vi "Calculate Points of Line without diagonal.vi"(8 "Yf":i32, 9 "Yi":i32, 10 "Xf":i32, 11 "Xi":i32) -> (2 "Y Points":i32[](array[numeric]), 3 "X Points":i32[](array[numeric]))   [LabVIEW 2019, in "Day 5.lvlib"]
uses:
  Day 5.lvlib
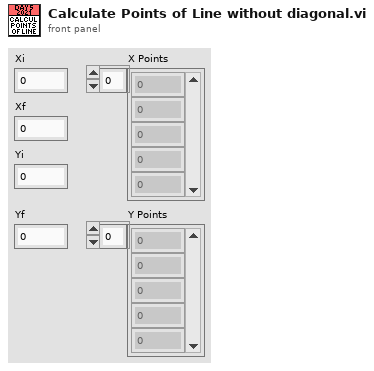
[diagram p1: front panel]
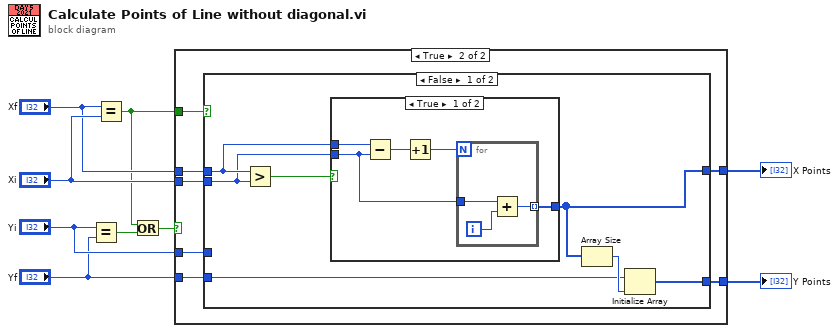
[diagram p0: block diagram]
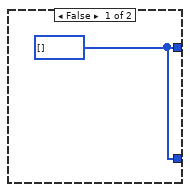
[diagram p2: hidden frame]
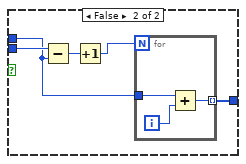
[diagram p3: hidden frame]
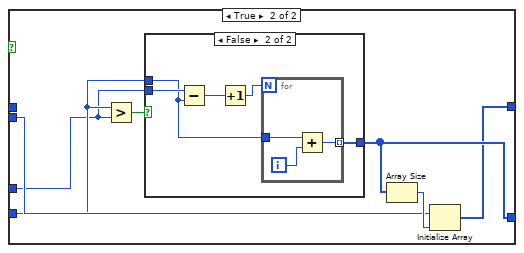
[diagram p4: hidden frame]
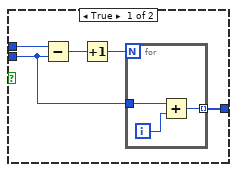
[diagram p5: hidden frame]
diagram:
  n1 = Equal?(x="Yi", y="Yf") -> (x = y?=w2:bool)
  n2 = Equal?(x="Xf", y="Xi") -> (x = y?=w3:bool)
  n3 = Or(x=w3, y=w2) -> (x .or. y?=w1:bool)
  n4 = case shown="True" w1 {
    tunnel: w3 -> [_ w17]
    tunnel: "Xi" -> [_ w16]
    tunnel: "Xf" -> [_ w15]
    tunnel: "Yi" -> [_ w14]
    tunnel: "Yf" -> [_ w13]
    tunnel: [w10 w12] -> w7
    tunnel: [w10 w11] -> w6
    frame False {
      w10 = i32[] []
    }
    frame True {
      n5 = case shown="False" w17 {
        tunnel: w16 -> [w22 w43]
        tunnel: w15 -> [w23 _]
        tunnel: w14 -> [_ w41]
        tunnel: w13 -> [w20 w42]
        tunnel: [w18 w46] -> w12
        tunnel: [w19 w44] -> w11
        frame False {
          n6 = Greater?(x=w23, y=w22) -> (0:w24:bool)
          n7 = case shown="True" w24 {
            tunnel: w23 -> [w29 w35]
            tunnel: w22 -> [w28 w36]
            tunnel: [w27 w37] -> w19
            frame True {
              n8 = Subtract(x=w29, y=w28) -> (x-y=w26:i32)
              n9 = Increment(x=w26) -> (x+1=w25:i32)
              n10 = for {
                N: w25 -> [_]
                tunnel: w28 -> [w32]
                tunnel: [w30] -> w27 mode=indexing
                i -> [w31]
                n11 = Add(x=w32, y=w31) -> (x+y=w30:i32)
              }
            }
            frame False {
              n12 = Subtract(x=w36, y=w35) -> (x-y=w34:i32)
              n13 = Increment(x=w34) -> (x+1=w33:i32)
              n14 = for {
                N: w33 -> [_]
                tunnel: w35 -> [w40]
                tunnel: [w38] -> w37 mode=indexing
                i -> [w39]
                n15 = Add(x=w40, y=w39) -> (x+y=w38:i32)
              }
            }
          }
          n16 = Array Size(array=w19) -> (size(s)=w21:i32)
          n17 = Initialize Array(w20, w21) -> (w18:i32[])
        }
        frame True {
          n18 = Greater?(x=w42, y=w41) -> (0:w47:bool)
          n19 = case shown="False" w47 {
            tunnel: w42 -> [w52 w58]
            tunnel: w41 -> [w51 w59]
            tunnel: [w50 w60] -> w46
            frame True {
              n20 = Subtract(x=w52, y=w51) -> (x-y=w49:i32)
              n21 = Increment(x=w49) -> (x+1=w48:i32)
              n22 = for {
                N: w48 -> [_]
                tunnel: w51 -> [w55]
                tunnel: [w53] -> w50 mode=indexing
                i -> [w54]
                n23 = Add(x=w55, y=w54) -> (x+y=w53:i32)
              }
            }
            frame False {
              n24 = Subtract(x=w59, y=w58) -> (x-y=w57:i32)
              n25 = Increment(x=w57) -> (x+1=w56:i32)
              n26 = for {
                N: w56 -> [_]
                tunnel: w58 -> [w63]
                tunnel: [w61] -> w60 mode=indexing
                i -> [w62]
                n27 = Add(x=w63, y=w62) -> (x+y=w61:i32)
              }
            }
          }
          n28 = Array Size(array=w46) -> (size(s)=w45:i32)
          n29 = Initialize Array(w43, w45) -> (w44:i32[])
        }
      }
    }
  }
  "Y Points" <- w7
  "X Points" <- w6
